vi "Resample (single).vi"(8 "error in (no error)":errorcluster, 9 "t0":dbl=-inf format="%.2p", 10 "dt":dbl=1.0 format="%.2p", 11 "XY-data":cluster{"X-array":dbl[], "Y-array":dbl[]} {"Y-array" format="%.2p"; "X-array" format="%.2p"}) -> (0 "error out":errorcluster, 3 "Resampled XY-data out":cluster{"X-array":dbl[], "Y-array":dbl[]} {"Y-array" format="%.2p"; "X-array" format="%.2p"})   [LabVIEW 2016, in "xy_utilities.lvlib"]
doc: "Resamples <b>XY-data</b> according to user-defined <b>dt</b> and <b>t0</b>. This VI is a wrapper for NI_MAPro.lvlib:Resample Waveforms (single shot).vi.\n\nWire data to the data input to determine the polymorphic instance to use or manually select the instance."
uses:
  xy_utilities.lvlib
  <vilib>/measure/maresamp.llb/Resample Pair of Arrays (single shot).vi
  <vilib>/measure/NI_MAPro.lvlib
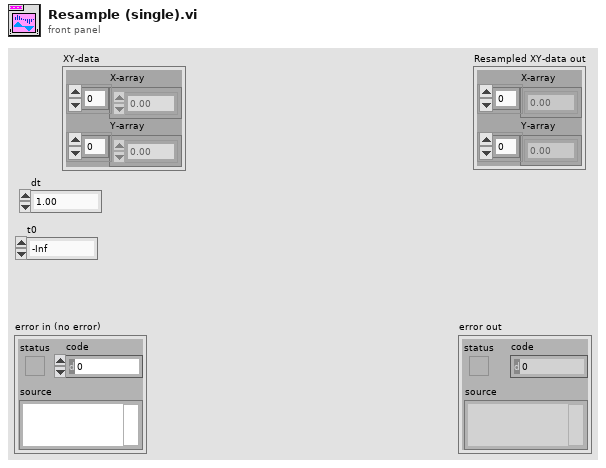
[diagram p1: front panel]
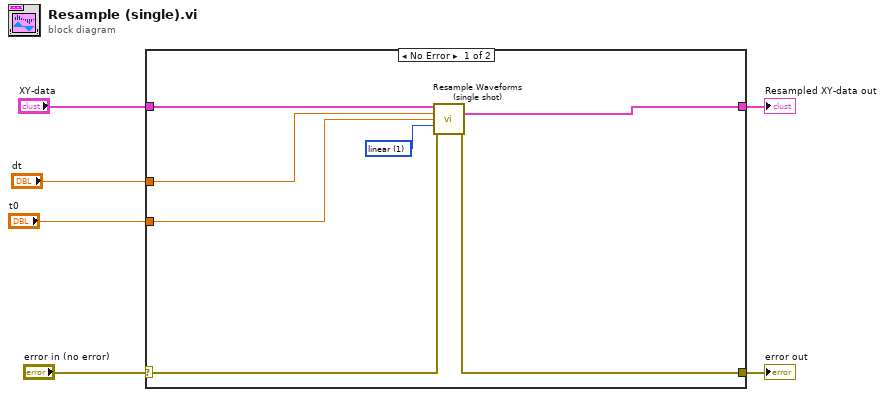
[diagram p0: block diagram]
diagram:
  n1 = case shown="No Error" "error in (no error)" {
    selector: "error in (no error)" -> [w12 w15]
    tunnel: [w11 w15] -> w5
    tunnel: "XY-data" -> [w13 w14]
    tunnel: [w10 w14] -> w3
    tunnel: "dt" -> [w9 _]
    tunnel: "t0" -> [w8 _]
    frame No Error {
      w7 = u16 1 items=["coerce", "linear", "spline", "FIR filter"] ("interpolation mode")
      n2 = call-poly <vilib>:"Resample Waveforms (single shot).vi"("XY-data in"=w13, "dt"=w9, "t0"=w8, "interpolation mode"=w7, "error in (no error)"=w12) -> ("XY-data out"=w10:cluster{"X-array":dbl[], "Y-array":dbl[]}, "error out"=w11:errorcluster)  [unwired: 6 in, 3 out]
    }
    frame Error {
    }
  }
  "error out" <- w5
  "Resampled XY-data out" <- w3
